vi "Scan Multi Bias (With Setpoint Control-REVISED).vi"(0 "Series Name":string="ScanMultiBias_" caption="Serie name", 1 "Avoid zero threshold (V)":dbl=0.004999999888241291 format="%#_13g", 3 "Pre-scan time [ms]":dbl, 5 "Number of scans":u8=5, 9 "Bias":sgl[](array[numeric])=[0.0, 0.0], 11 "Setpoint":sgl[](array[numeric])=[0.0, 0.0], 12 "Auto save":bool=TRUE) -> (4 "Scan":u8 caption="Current scan", 15 "Error out":errorcluster)   [LabVIEW 2025]
doc: "This example performs multiple image scans, increasing the bias voltage after each scan.\n\n- Nanonis Programming Interface -"
uses:
  <userlib>/Nanonis Prog Interface V5e/Nanonis Prog Interface.lvlib
panel:
  in  "Machine name (local machine IP)":string
  # "Example program for the Nanonis SPM Control software programming interface\n(see diagram)."
  # "SET ALL PARAMETERS FOR # OF SCAN (I.E. 50 scans = 50 Parameters"
  # "This example performs multiple image scans, increasing the bias voltage after each scan."
  # "Change Bias based on iteration of scan"
  # "Change Setpoint based on iteration of scan"
  # "Set to 0.05M to go from -100 mV to 100 mV"
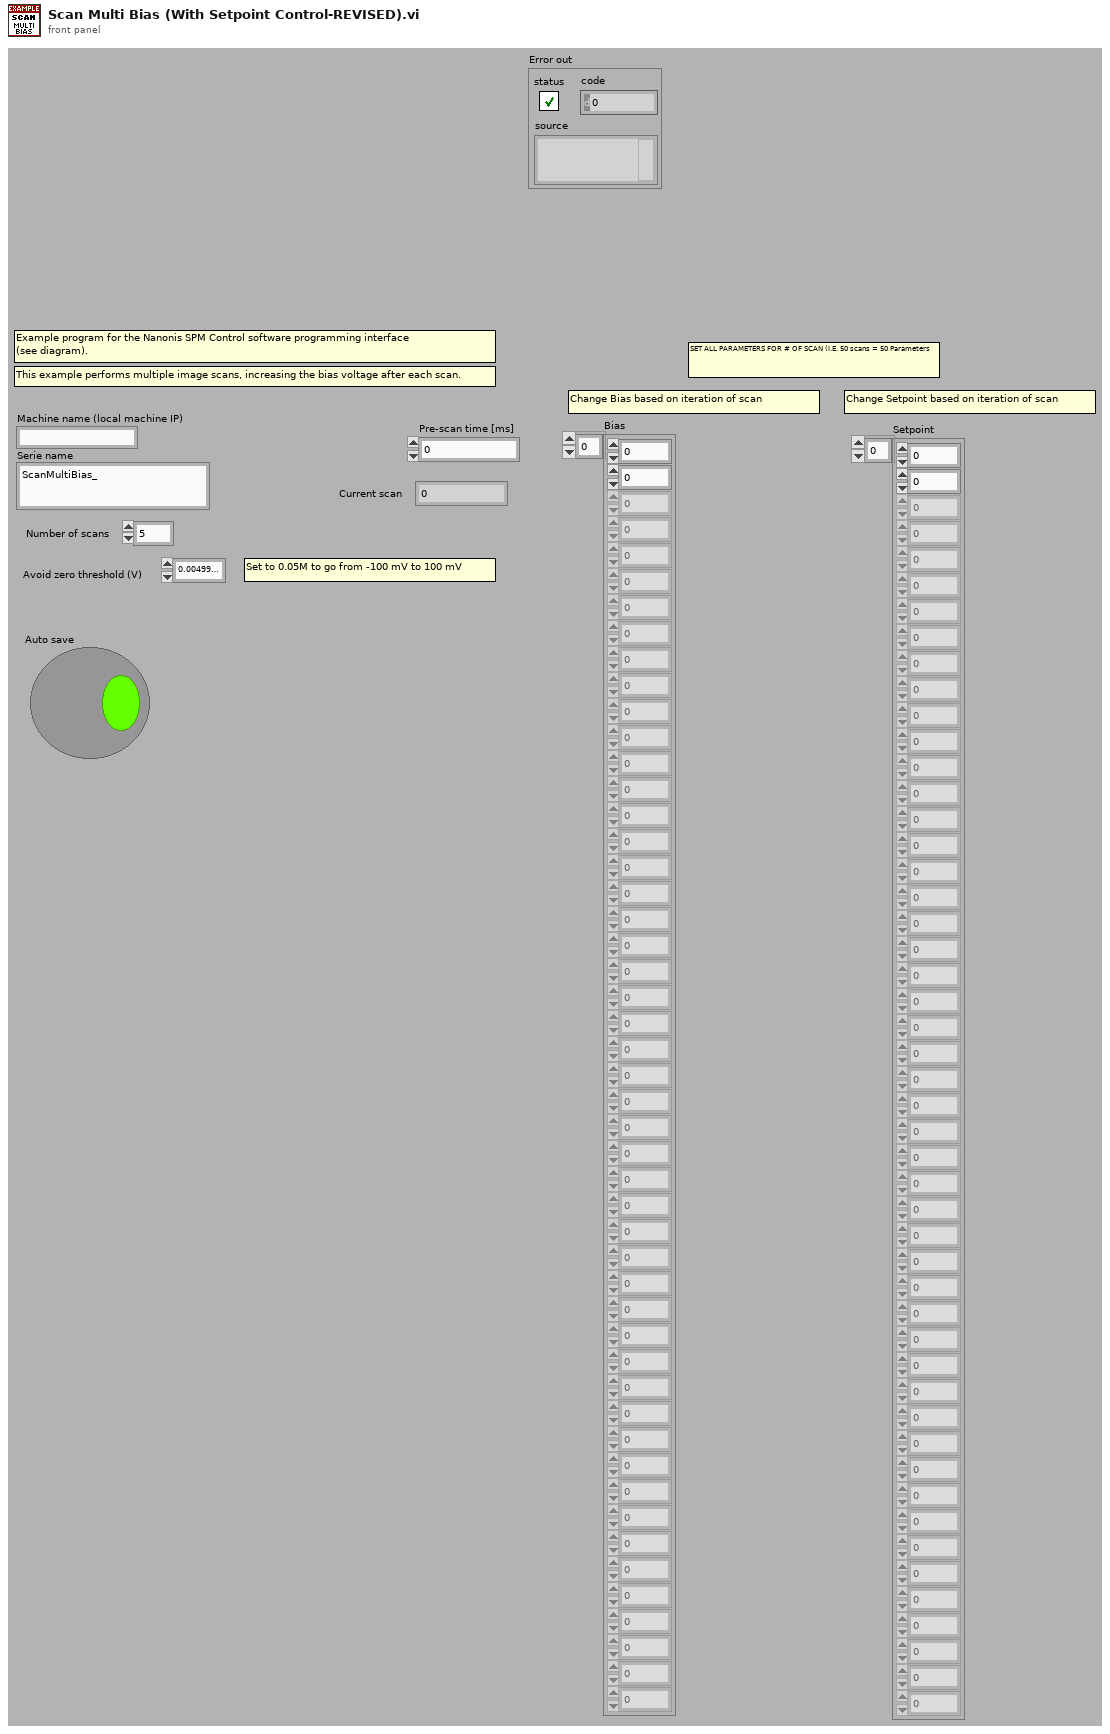
[diagram p1: front panel]
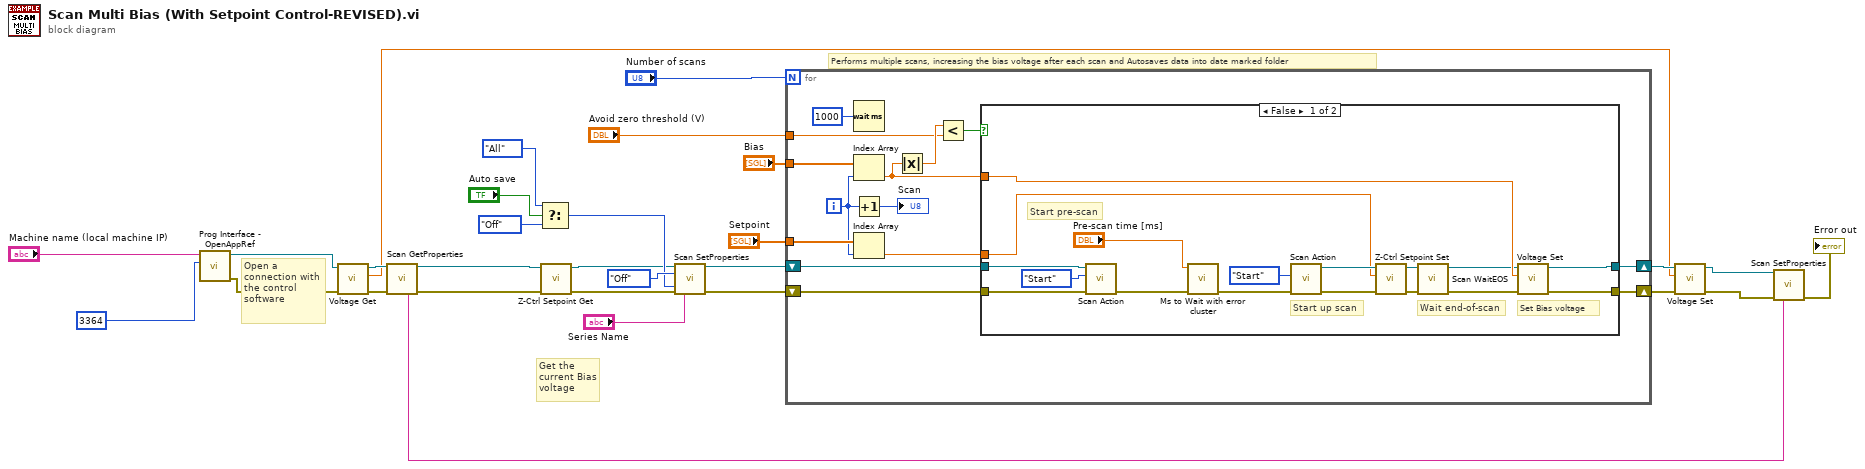
[diagram p0: block diagram]
diagram:
  # "Open a connection with the control\nsoftware"
  # "Performs multiple scans, increasing the bias voltage after each scan and Autosaves data into date marked folder"
  # "Get the current Bias voltage"
  n1 = call <userlib>:"Prog Interface - OpenAppRef.vi"("Port number (3364)"=u32 3364, "Machine name (local machine IP)"="Machine name (local machine IP)") -> ("Error out"=w29:errorcluster, "Application reference"=w21:refnum<vi>)  [unwired: 4 in]
  n2 = call <userlib>:"Voltage Get.vi"("error in (no error)"=w29, "Application ref in"=w21) -> ("error out"=w16:errorcluster, "Bias (V)"=w6:sgl, "Application ref out"=w17:refnum<vi>)  [unwired: 7 in]
  n3 = call <userlib>:"Scan GetProperties.vi"("Application ref in"=w17, "Error in (no error)"=w16) -> ("Application ref out"=w12:refnum<vi>, "Serie name"=w15:string, "Error out"=w13:errorcluster)  [unwired: 5 in, 6 out]
  n4 = Select(t=enum16{"No change", "All", "Next", "Off"}."All" ("Auto save"), s="Auto save", f=enum16{"No change", "All", "Next", "Off"}."Off" ("Auto save")) -> (s? t:f=w22:enum16{"No change", "All", "Next", "Off"})
  n5 = call <userlib>:"Z-Ctrl Setpoint Get.vi"("error in (no error)"=w13, "Application ref in"=w12) -> ("error out"=w10:errorcluster, "Application ref out"=w11:refnum<vi>)  [unwired: 6 in, 1 out]
  n6 = call <userlib>:"Scan SetProperties.vi"("Application ref in"=w11, "Continuous scan"=enum16{"No change", "On", "Off"}."Off", "Auto save"=w22, "Error in (no error)"=w10, "Serie name"="Series Name") -> ("Application ref out"=w20:refnum<vi>, "Error out"=w28:errorcluster)  [unwired: 9 in]
  n7 = for {
    N: "Number of scans" -> [_]
    shift-right: [w38] -> w18
    shift-left: w28 -> [w43]
    shift-right: [w39] -> w19
    shift-left: w20 -> [w42]
    tunnel: "Avoid zero threshold (V)" -> [w37]
    tunnel: "Setpoint" -> [w36]
    tunnel: "Bias" -> [w33]
    i -> [w32]
    n8 = Wait (ms)(milliseconds to wait=u32 1000) -> ()  [unwired: 1 out]
    n9 = Index Array(array=w33, index=w32) -> (element=w31:sgl)
    n10 = Increment(x=w32) -> (x+1=→"Scan":i32)
    n11 = Index Array(array=w36, index=w32) -> (element=w35:sgl)
    n12 = Absolute Value(x=w31) -> (abs(x)=w41:sgl)
    n13 = Less?(x=w41, y=w37) -> (x < y?=w40:bool)
    n14 = case shown="False" w40 {
      tunnel: w43 -> [w60 w61]
      tunnel: w31 -> [w59 _]
      tunnel: w42 -> [w57 w62]
      tunnel: [w52 w62] -> w39
      tunnel: [w51 w61] -> w38
      tunnel: w35 -> [w46 _]
      frame False {
        # "Start up scan"
        # "Set Bias voltage"
        # "Wait end-of-scan"
        # "Start pre-scan"
        n15 = call <userlib>:"Scan Action.vi"("error in (no error)"=w60, "Scan action (Start)"=enum16{"Start", "Stop", "Pause", "Resume"}."Start" ("Scan action"), "Application ref in"=w57) -> ("error out"=w55:errorcluster)  [unwired: 6 in, 1 out]
        n16 = call <userlib>:"Ms to Wait with error cluster.vi"("error in (no error)"=w55, "milliseconds to wait"="Pre-scan time [ms]") -> ("error out"=w54:errorcluster)  [unwired: 4 in, 1 out]
        n17 = call <userlib>:"Scan Action.vi"("error in (no error)"=w54, "Scan action (Start)"=enum16{"Start", "Stop", "Pause", "Resume"}."Start" ("Scan action")) -> ("error out"=w50:errorcluster, "Application ref out"=w47:refnum<vi>)  [unwired: 7 in]
        n18 = call <userlib>:"Z-Ctrl Setpoint Set.vi"("error in (no error)"=w50, "Z Controller setpoint"=w46, "Application ref in"=w47) -> ("error out"=w49:errorcluster, "Application ref out"=w48:refnum<vi>)  [unwired: 7 in]
        n19 = call <userlib>:"Scan WaitEOS.vi"("error in (no error)"=w49, "Application ref in"=w48) -> ("error out"=w44:errorcluster, "Application ref out"=w45:refnum<vi>)  [unwired: 5 in, 2 out]
        n20 = call <userlib>:"Voltage Set.vi"("Error in (no error)"=w44, "Bias (V)"=w59, "Application ref in"=w45) -> ("Error out"=w51:errorcluster, "Application ref out"=w52:refnum<vi>)  [unwired: 7 in]
      }
      frame True {
      }
    }
  }
  n21 = call <userlib>:"Voltage Set.vi"("Error in (no error)"=w18, "Bias (V)"=w6, "Application ref in"=w19) -> ("Error out"=w8:errorcluster, "Application ref out"=w7:refnum<vi>)  [unwired: 7 in]
  n22 = call <userlib>:"Scan SetProperties.vi"("Application ref in"=w7, "Error in (no error)"=w8, "Serie name"=w15) -> ("Error out"=→"Error out":errorcluster)  [unwired: 11 in, 1 out]
